vi "singleActionGUI_v12.vi"() -> ()   [LabVIEW 2012]
panel:
  in  "?":bool
  in  "?":bool
  out "Max speed (mm/s):":dbl
  in  "?":dbl
  out "Max extension (mm):":dbl
  out "Current position (mm):":dbl
  out "Max force (N):":dbl
  out "Current force (N):":dbl
  in  "?":dbl
  in  "?":bool
  in  "?":bool
  in  "?":bool
  in  "?":enum32{"", ""}(radio)
  out "Max speed (mm):":dbl
  out "Step size (mm):":dbl
  out "Max position (mm):":dbl
  out "Current position (mm):":dbl
  in  "Position (mm)":dbl
  in  "?":bool
  in  "?":bool
  in  "?":bool
  in  "?":bool
  in  "?":bool
  in  "?":enum32{"", ""}(radio)
  in  "Speed (mm/s)":dbl=0.1 min=0.1 step=0.5 format="%.2g"
  # "Stage panel"
  # "Roller panel"
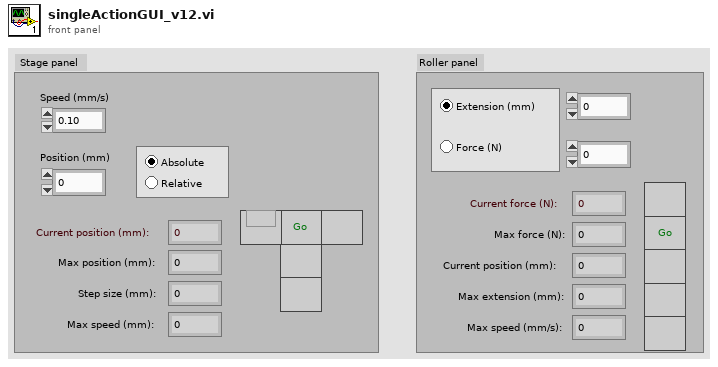
[diagram p1: front panel]
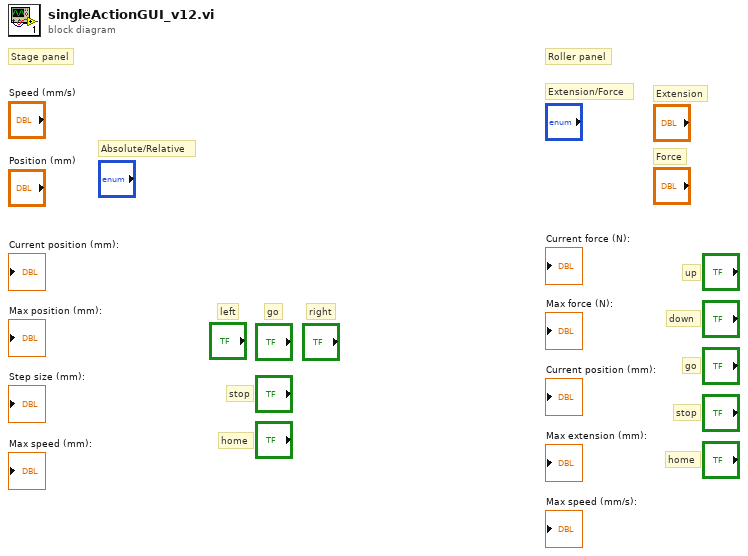
[diagram p0: block diagram]
diagram:
  # "Force"
  # "Extension"
  # "Extension/Force"
  # "Absolute/Relative"
  # "home"
  # "stop"
  # "right"
  # "left"
  # "go"
  # "home"
  # "stop"
  # "go"
  # "down"
  # "up"
  # "Roller panel"
  # "Stage panel"
